vi "Calculate Friction Force.vi"(8 "error in":errorcluster, 10 "Friction in":refnum<class "Friction.lvclass">, 11 "Mover in":refnum<class "Mover.lvclass">) -> (0 "error out":errorcluster, 2 "Friction Force out":refnum<class "PVector.lvclass">, 3 "Mover out":refnum<class "Mover.lvclass">)   [LabVIEW 2016, in "Mover.lvclass"]
uses:
  Mover.lvclass
  Forces/Friction/Friction.lvclass
  PVector/PVector.lvclass
  Mover.lvclass/Mover.ctl
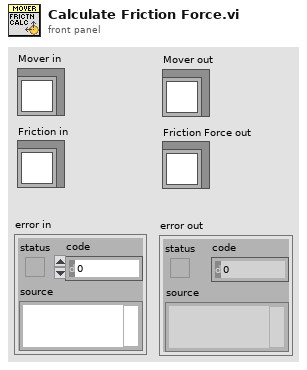
[diagram p1: front panel]
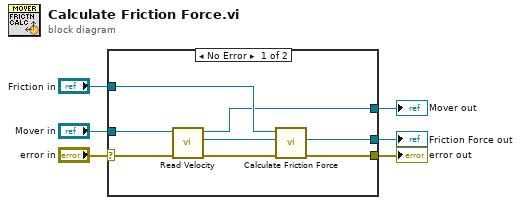
[diagram p0: block diagram]
diagram:
  n1 = case shown="No Error" "error in" {
    selector: "error in" -> [w13 w16]
    tunnel: [w10 w16] -> w5
    tunnel: [w7 w15] -> w3
    tunnel: "Mover in" -> [w14 w15]
    tunnel: "Friction in" -> [w9 _]
    tunnel: [w8 _] -> w1
    frame No Error {
      n2 = call "Read Velocity.vi"("error in"=w13, "Mover in"=w14) -> ("error out"=w11:errorcluster, "Velocity PVector"=w12:refnum<class "PVector.lvclass">, "Mover out"=w7:refnum<class "Mover.lvclass">)  [unwired: 7 in]
      n3 = call "Calculate Friction Force.vi"("error in"=w11, "Mover Velocity in"=w12, "Friction in"=w9) -> ("error out"=w10:errorcluster, "Friction Force Out"=w8:refnum<class "PVector.lvclass">)  [unwired: 6 in, 1 out]
    }
    frame Error {
    }
  }
  "error out" <- w5
  "Mover out" <- w3
  "Friction Force out" <- w1
